vi "startCamera.vi"(8 "error in (no error)":errorcluster, 10 "camera":string, 11 "BECHWCBasic in":refnum<class "BECHWCBasic.lvclass">) -> (0 "error out":errorcluster, 3 "BECHWCBasic out":refnum<class "BECHWCBasic.lvclass">)   [LabVIEW 2009, in "Hardware.lvlib" / "HWControllers.lvlib" / "BECHWCBasic.lvclass"]
uses:
  BECHWCBasic.lvclass
  BECHWCBasic.lvclass/BECHWCBasic.ctl
  IntegrationManagement/CameraManager.lvclass
  HWController.lvclass
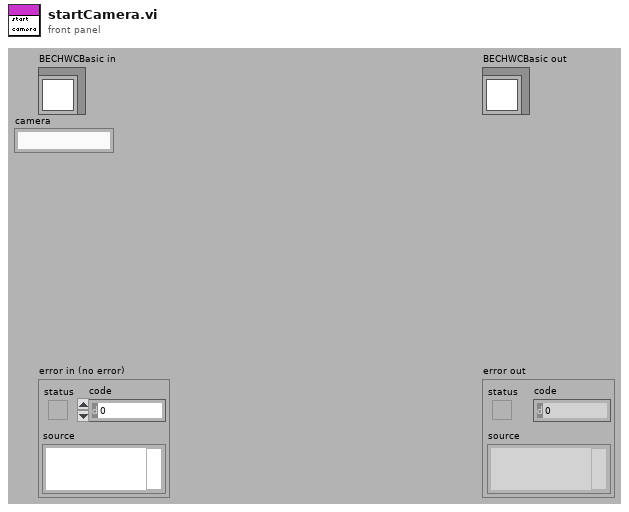
[diagram p1: front panel]
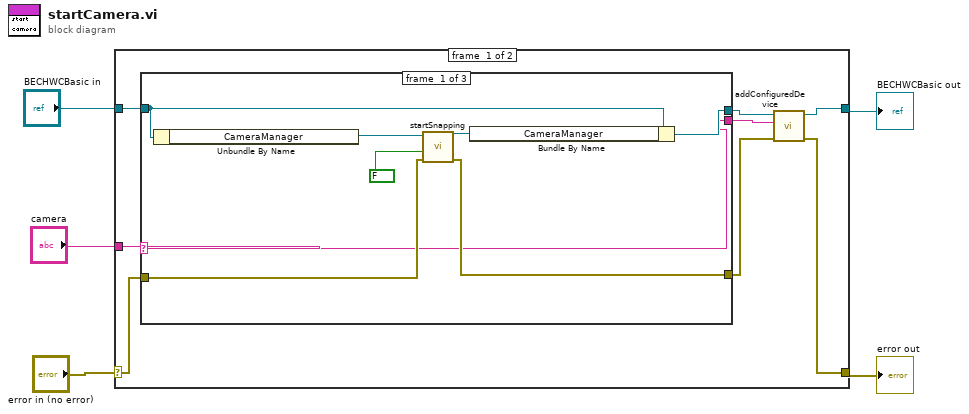
[diagram p0: block diagram]
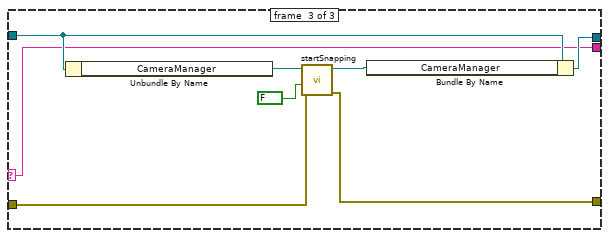
[diagram p3: hidden frame]
diagram:
  n1 = case shown="No Error" "error in (no error)" {
    selector: "error in (no error)" -> [w11 w33]
    tunnel: [w7 w33] -> w4
    tunnel: [w6 w32] -> w2
    tunnel: "BECHWCBasic in" -> [w12 w32]
    tunnel: "camera" -> [w13 _]
    frame #0 {
      n2 = case shown="\"AndorIKon\"" w13 {
        selector: w13 -> [w14 _ w24]
        tunnel: w12 -> [w17 w23 w30]
        tunnel: w11 -> [w16 w22 w27]
        tunnel: [w15 w22 w26] -> w8
        tunnel: [w18 w23 w25] -> w10
        tunnel: [w14 _ w24] -> w9
        frame #0 {
          n3 = Unbundle By Name(w17) -> ("CameraManager"=w20:refnum<class "CameraManager.lvclass">)
          n4 = call "startSnapping.vi"("error in (no error)"=w16, "releaseWhenReady"=FALSE, "CameraManager in"=w20) -> ("error out"=w15:errorcluster, "CameraManager out"=w19:refnum<class "CameraManager.lvclass">)  [unwired: 7 in]
          n5 = Bundle By Name(cluster=w17, "CameraManager"=w19) -> (w18:refnum<class "BECHWCBasic.lvclass">)
        }
        frame #1 {
        }
        frame #2 {
          n6 = Unbundle By Name(w30) -> ("CameraManager"=w31:refnum<class "CameraManager.lvclass">)
          n7 = call "startSnapping.vi"("error in (no error)"=w27, "releaseWhenReady"=FALSE, "CameraManager in"=w31) -> ("error out"=w26:errorcluster, "CameraManager out"=w29:refnum<class "CameraManager.lvclass">)  [unwired: 7 in]
          n8 = Bundle By Name(cluster=w30, "CameraManager"=w29) -> (w25:refnum<class "BECHWCBasic.lvclass">)
        }
      }
      n9 = call "addConfiguredDevice.vi"("error in (no error)"=w8, "deviceName"=w9, "HWController in"=w10) -> ("error out"=w7:errorcluster, "HWController out"=w6:refnum<class "BECHWCBasic.lvclass">)  [unwired: 7 in]
    }
    frame #1 {
    }
  }
  "error out" <- w4
  "BECHWCBasic out" <- w2
